vi "_PC_D999_Display_Data.vi"(7 "Listbox":refnum<vi>, 8 "error in":errorcluster) -> (0 "error out":errorcluster)   [LabVIEW 2018]
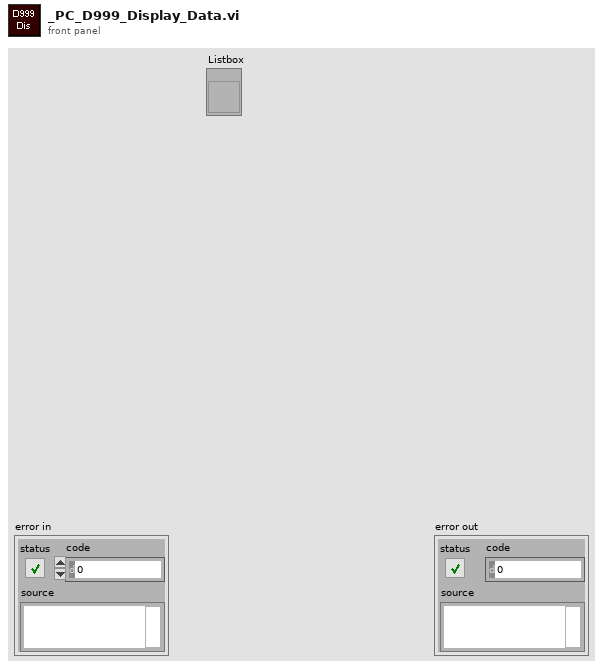
[diagram p1: front panel]
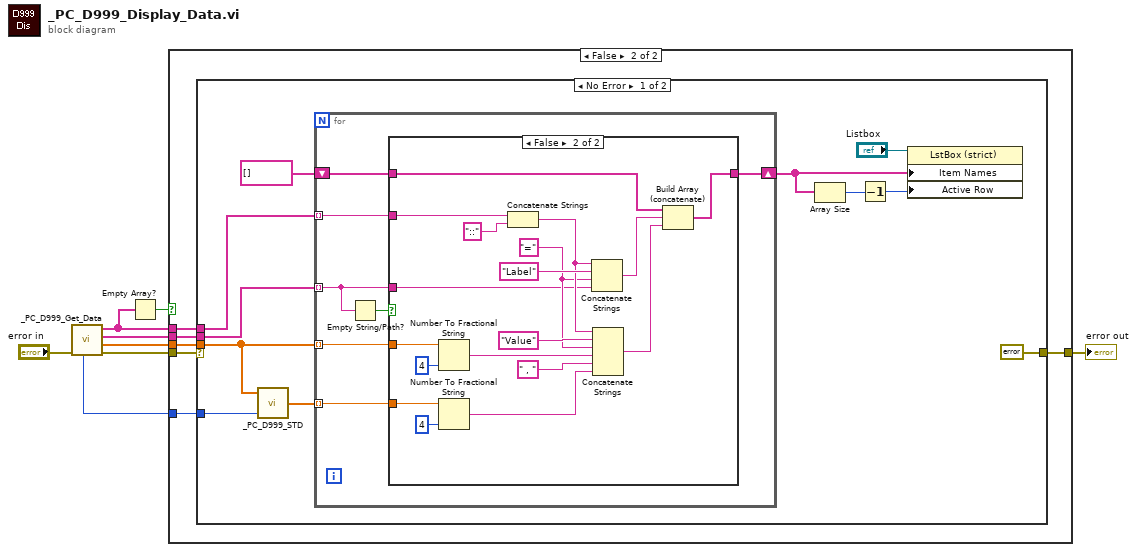
[diagram p0: block diagram]
diagram:
  n1 = call "_PC_D999_Get_Data.vi"("error in (no error)"="error in") -> ("error IO"=w7:errorcluster, "Value Array"=w2:dbl[], "Label array"=w4:string[], "Port array"=w3:string[], "index"=w1:u8)  [unwired: 5 in, 1 out]
  n2 = Empty Array?(array=w3) -> (empty?=w5:bool)
  n3 = case shown="False" w5 {
    tunnel: [_ w14] -> w8
    tunnel: w1 -> [_ w13]
    tunnel: w7 -> [_ w12]
    tunnel: w4 -> [_ w11]
    tunnel: w3 -> [_ w10]
    tunnel: w2 -> [_ w9]
    frame True {
    }
    frame False {
      n4 = case shown="No Error" w12 {
        selector: w12 -> [_ w52]
        tunnel: [errorcluster {"status"=FALSE, "code"=0, "source"=""} ("error out") w52] -> w14
        tunnel: w13 -> [w20 _]
        tunnel: w11 -> [w16 _]
        tunnel: w10 -> [w17 _]
        tunnel: w9 -> [w15 _]
        frame No Error {
          n5 = call "_PC_D999_STD.vi"("index (row)"=w20, "new element/subarray"=w15) -> ("STD"=w18:dbl[])  [unwired: 1 in]
          n6 = for {
            shift-right: [w32] -> w19
            shift-left: string[] [] -> [w29]
            tunnel: w15 -> [w31] mode=indexing
            tunnel: w18 -> [w30] mode=indexing
            tunnel: w16 -> [w27] mode=indexing
            tunnel: w17 -> [w26] mode=indexing
            n7 = Empty String/Path?(string/path=w27) -> (empty?=w28:bool)
            n8 = case shown="False" w28 {
              tunnel: [w33 w51] -> w32
              tunnel: w31 -> [_ w45]
              tunnel: w30 -> [_ w42]
              tunnel: w29 -> [w33 w38]
              tunnel: w27 -> [_ w37]
              tunnel: w26 -> [_ w34]
              frame True {
              }
              frame False {
                w39 = "="
                n9 = Number To Fractional String(number=w45, precision (6)=i16 4) -> (F-format string=w44:string)  [unwired: 2 in]
                n10 = Number To Fractional String(number=w42, precision (6)=i16 4) -> (F-format string=w35:string)  [unwired: 2 in]
                n11 = Concatenate Strings(w34, "::") -> (w40:string)
                n12 = Concatenate Strings(w40, "Label" ("string"), w39, w37) -> (w49:string)
                n13 = Concatenate Strings(w40, "Value" ("string"), w39, w44, " , " ("string"), w35) -> (w48:string)
                n14 = Build Array (concatenate)(w38, w49, w48) -> (w51:string[])
              }
            }
          }
          n15 = Array Size(array=w19) -> (size(s)=w24:i32)
          n16 = Decrement(x=w24) -> (x-1=w25:i32)
          n17 = property class="LstBox (strict)"(reference="Listbox", "Item Names"=w19, "Active Row"=w25) -> ()  [unwired: 1 in, 2 out]
        }
        frame Error {
        }
      }
    }
  }
  "error out" <- w8
